vi "Set Control Reference.vi"(8 "error in (no error)":errorcluster, 10 "Control Reference":refnum<vi>, 11 "Item Configuration in":refnum<class "Item Configuration.lvclass">) -> (0 "error out":errorcluster, 3 "Item Configuration out":refnum<class "Item Configuration.lvclass">)   [LabVIEW 2013, in "Item Configuration.lvlib" / "Item Configuration.lvclass"]
uses:
  Item Configuration.lvclass
  Item Configuration.lvclass/Item Configuration.ctl
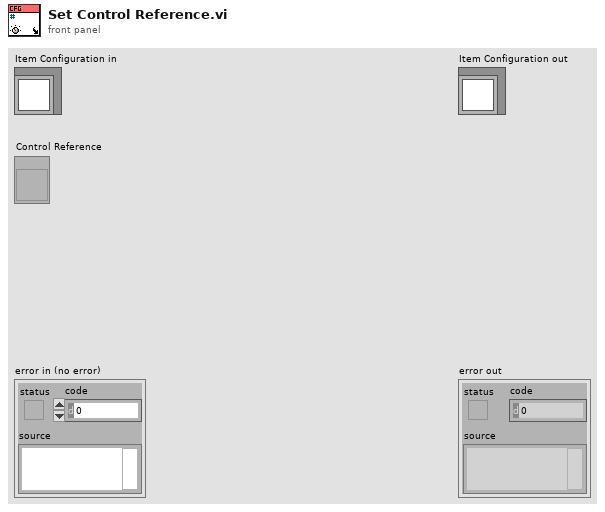
[diagram p1: front panel]
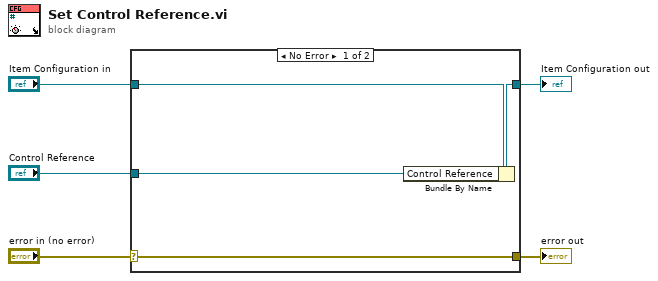
[diagram p0: block diagram]
diagram:
  n1 = case shown="No Error" "error in (no error)" {
    selector: "error in (no error)" -> [w9 w10]
    tunnel: [w9 w10] -> w4
    tunnel: [w7 w11] -> w2
    tunnel: "Item Configuration in" -> [w8 w11]
    tunnel: "Control Reference" -> [w6 _]
    frame No Error {
      n2 = Bundle By Name(cluster=w8, "Control Reference"=w6) -> (w7:refnum<class "Item Configuration.lvclass">)
    }
    frame Error {
    }
  }
  "error out" <- w4
  "Item Configuration out" <- w2
